vi "SemmiColonStringToArray.vi"(11 "String":string) -> (3 "Array":string[](array[string]))   [LabVIEW 2013, in "main.lvlib"]
uses:
  main.lvlib
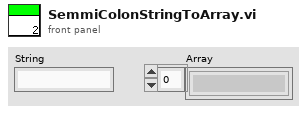
[diagram p1: front panel]
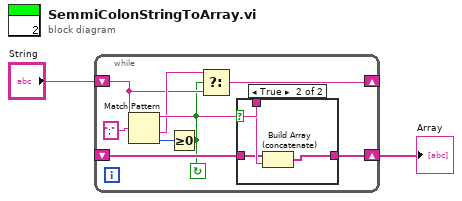
[diagram p0: block diagram]
diagram:
  n1 = while {
    shift-right: [w9] -> _
    shift-left: "String" -> [w4]
    shift-right: [w6] -> w1
    shift-left: _ -> [w7]
    stop <- w3 continue-if-true
    n2 = Match Pattern(string=w4, regular expression=";") -> (before substring=w8:string, after substring=w5:string, offset past match=w10:i32)  [unwired: 2 out]
    n3 = Greater Or Equal To 0?(x=w10) -> (x >= 0?=w3:bool)
    n4 = Select(t=w5, s=w3, f=w4) -> (s? t:f=w9:string)
    n5 = case shown="True" w3 {
      tunnel: w8 -> [_ w15]
      tunnel: w7 -> [w12 w14]
      tunnel: [w12 w13] -> w6
      frame False {
      }
      frame True {
        n6 = Build Array (concatenate)(w14, w15) -> (w13:string[])
      }
    }
  }
  "Array" <- w1
